vi "Read DAT.vi"(6 "header length":i32=11, 8 "error in (no error)":errorcluster, 11 "File Path":path) -> (0 "error out":errorcluster, 2 "Data (Dictionary)":T1[](array[typedef]), 4 "Notes":string)   [LabVIEW 2016, in "LV-Data.DAT.lvclass"]
uses:
  LV-Data.DAT.lvclass
  LV-Data/Typedefs/Dictionary--cluster.ctl
  <vilib>/Utility/file.llb/Read Delimited Spreadsheet (string).vi
  LV-Data/LV-Data.lvclass
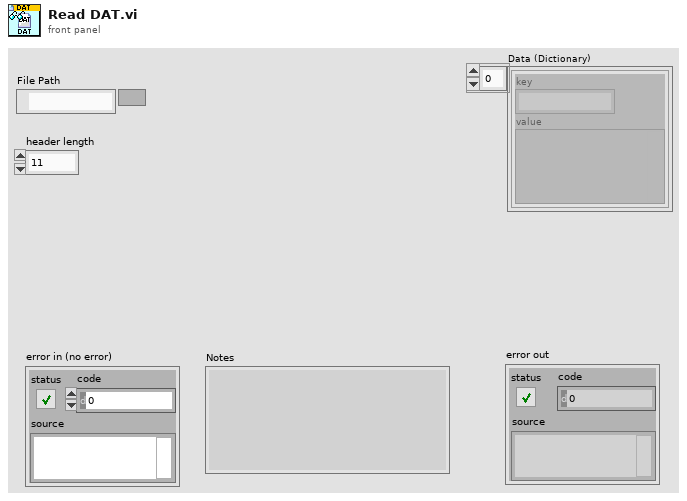
[diagram p1: front panel]
types:
  T1 = typedef "LV-Data.lvclass/Dictionary--cluster.ctl" = cluster{"key":string, "value":variant}
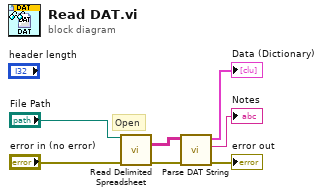
[diagram p0: block diagram]
diagram:
  # "Open"
  n1 = call-poly <vilib>:"Read Delimited Spreadsheet.vi"("file path (dialog if empty)"="File Path", "error in (no error)"="error in (no error)") -> ("all rows"=w6:string[][], "error out"=w2:errorcluster)  [unwired: 8 in, 4 out]
  n2 = call "Parse DAT String.vi"("error in (no error)"=w2, "spreadsheet string"=w6) -> ("error out"=→"error out":errorcluster, "Notes"=→"Notes":string, "Data (Dictionary)"=→"Data (Dictionary)":T1[])  [unwired: 7 in]
